vi "helper-snapshot.vi"(11 "RIO List":cluster{"Address":u8, "Connected":bool}[](array[cluster]) {"Address" format="%02d"}) -> (3 "Snapshot":T1[](array[typedef]) {"Dports" format="%08x"})   [LabVIEW 2024]
uses:
  controls/type-snapshot.ctl
  controls/enumVarCtrlIO.ctl
  controls/enum.io.type.ctl
  controls/enum.io.mode.ctl
  controls/IONode.ctl
  controls/type.address.ctl
  controls/typeXyPoint.ctl
  <vilib>/Utility/error.llb/Clear Errors.vi
  util.environment.vi
  util-address-parser.vi
  util.DO.ToString.vi
  Polymorphics/io.command-builder.vi
  Polymorphics/io.command-builder.DO.vi
  Polymorphics/io.command-builder.AI.vi
  Polymorphics/io.command-builder.DI.vi
  io.frame.vi
  io.visa.vi
  io.responseValidator.vi
  Polymorphics/io.command-parser.DI.vi
  Polymorphics/io.command-parser.AI.vi
  globals/globals-engine.vi
panel:
  in  "IO calib select":string(combo)
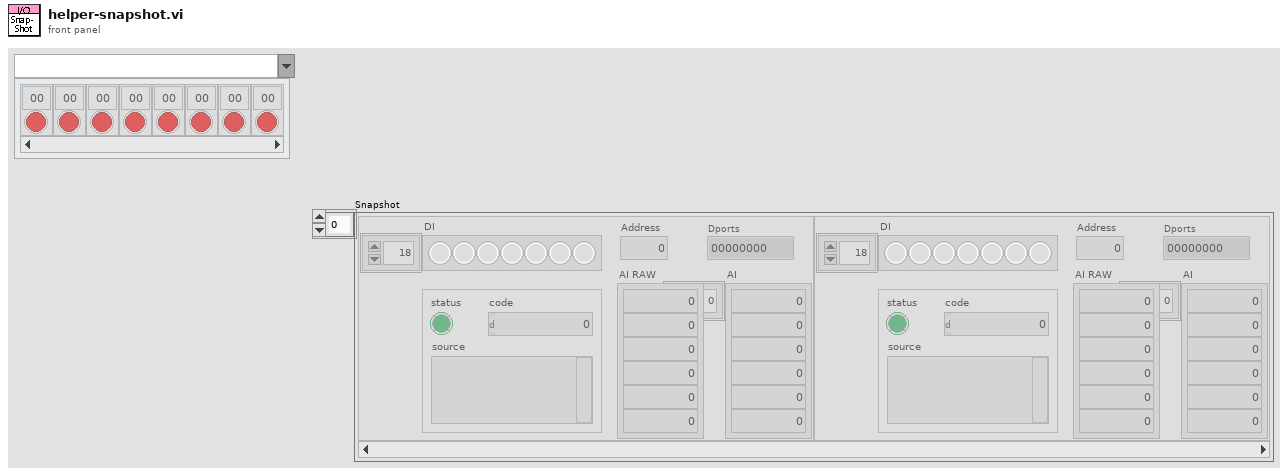
[diagram p1: front panel]
types:
  T1 = typedef "type-snapshot.ctl" = cluster{"Address":u8, "DI":bool[], "status":errorcluster, "AI":dbl[], "Dports":u32, "AI RAW":dbl[]}
  T2 = typedef "enumVarCtrlIO.ctl" = enum16{"IO Get By Key", "IO List Configs", "IO Add By Key", "IO Modify Value By Key", "IO Modify Calib By Key", "IO Modify ADDR By Key", "IO Modify Mode By Key", "IO Modify Type By Key", "IO Modify Name By Key", "IO Remove By Key", "IO Remove All"}
  T3 = typedef "IONode.ctl" = cluster{"ADDR":T4, "Label":string, "Type":T5, "Mode":T6, "Value":string, "Tags":string, "calibration":T7[]}
  T4 = typedef "type.address.ctl" = u16
  T5 = typedef "enum.io.type.ctl" = enum16{"Type", "DI", "DO", "AI", "AO", "VL", "BUF"}
  T6 = typedef "enum.io.mode.ctl" = enum16{"Mode", "RIO", "SIM"}
  T7 = typedef "typeXyPoint.ctl" = cluster{"X":dbl, "Y":dbl}
  T8 = cluster{"Device":u8, "Label":string, "Type":T5, "Mode":T6, "Tags":string}
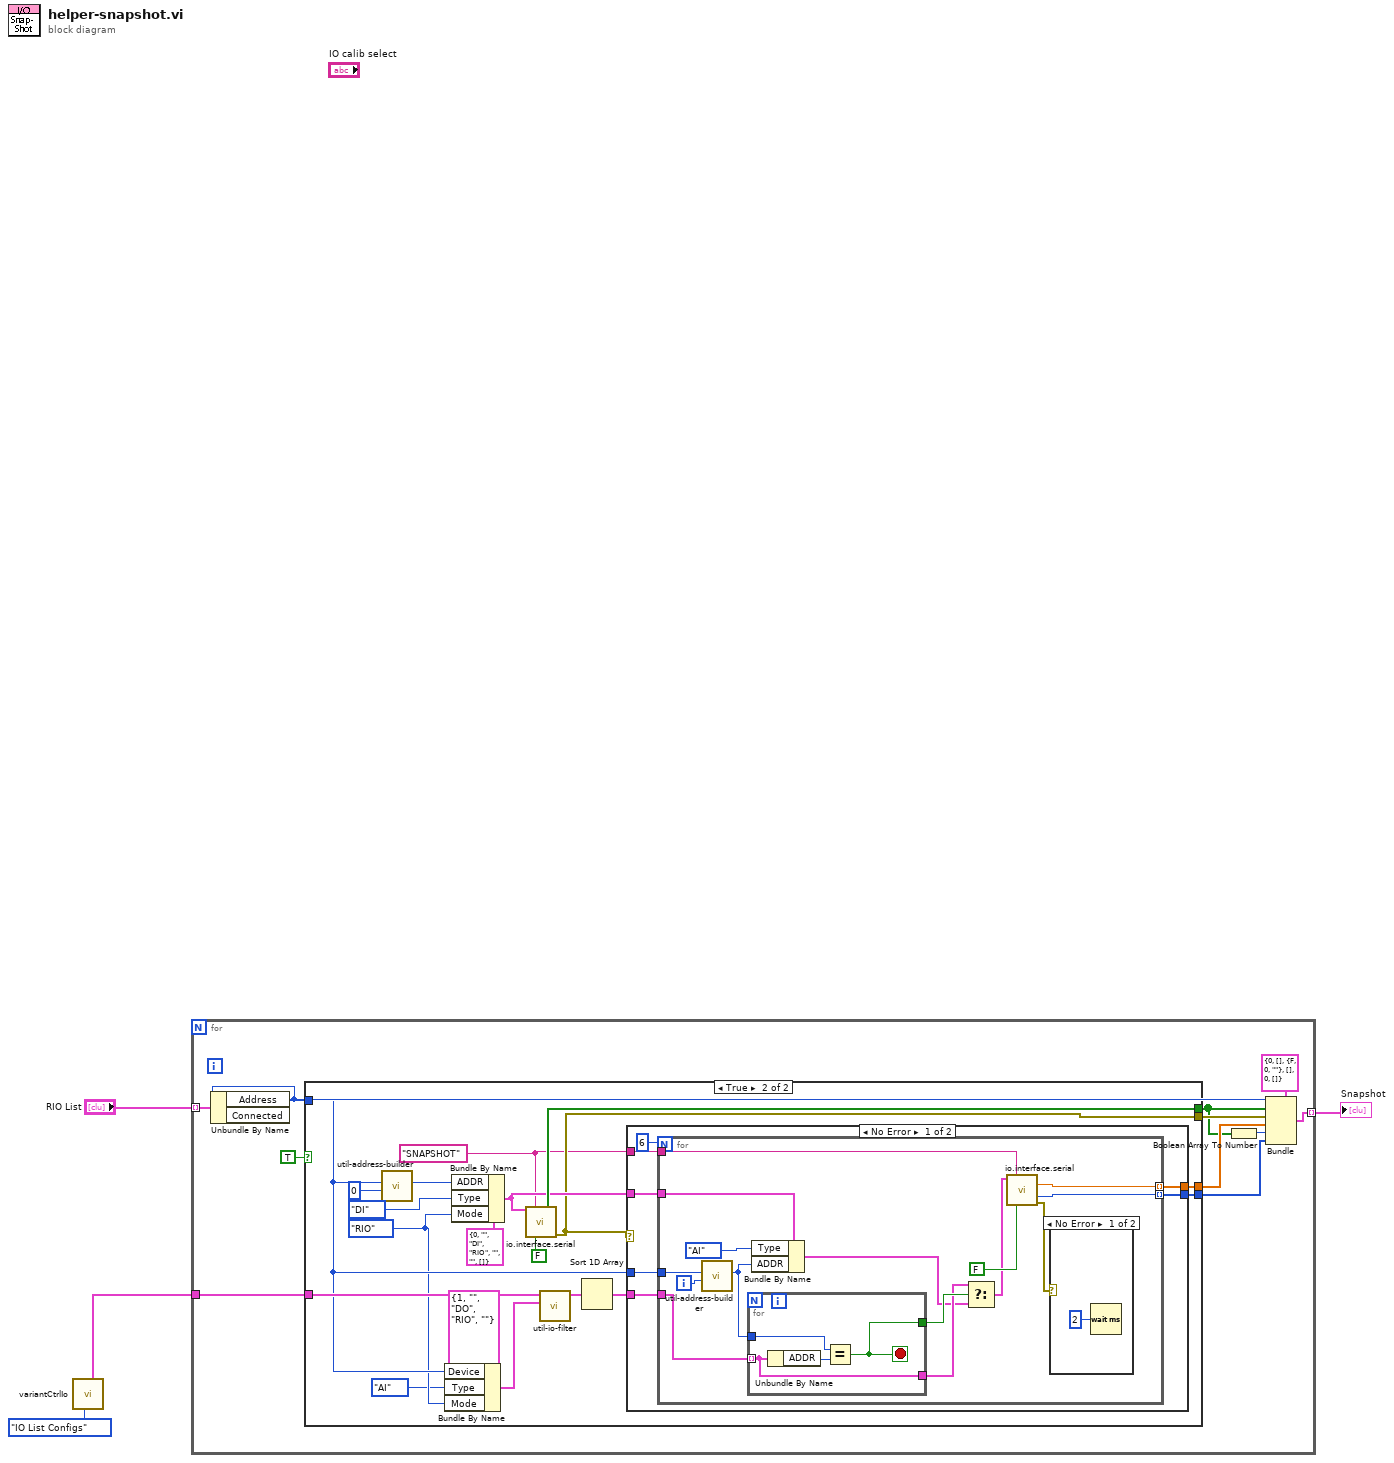
[diagram p0: block diagram]
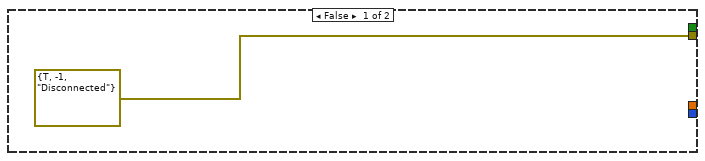
[diagram p2: hidden frame]
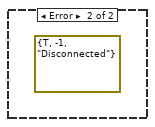
[diagram p4: hidden frame]
diagram:
  n1 = call "variantCtrlIo.vi"("menu (Get Param)"=enumVarCtrlIO."IO List Configs") -> ("IO Configs List"=w1:T3[])  [unwired: 6 in, 4 out]
  n2 = for {
    tunnel: [w15] -> w4 mode=indexing
    tunnel: "RIO List" -> [w12] mode=indexing
    tunnel: w1 -> [w10]
    n3 = Unbundle By Name(w12) -> ("Address"=w11:u8)  [unwired: 1 out]
    n4 = case shown="True" TRUE {
      tunnel: [_ w34] -> w8
      tunnel: [_ w31] -> w14
      tunnel: [errorcluster {"status"=TRUE, "code"=-1, "source"="Disconnected"} ("error out") w19] -> w13
      tunnel: w11 -> [_ w24]
      tunnel: w10 -> [_ w27]
      tunnel: [_ w17] -> w5
      frame False {
      }
      frame True {
        w18 = "SNAPSHOT" ("Caller")
        w23 = enum.io.mode."RIO" ("Mode")
        n5 = call "util-address-builder.vi"("Channel"=u8 0, "Device"=w24) -> ("ADDR"=w30:T4)  [unwired: 9 in]
        n6 = Bundle By Name(cluster=T8 {"Device"=1, "Label"="", "Type"=enum."DO", "Mode"=enum."RIO", "Tags"=""} ("IO Search Conf"), "Device"=w24, "Type"=enum.io.type."AI", "Mode"=w23) -> (w25:T8)
        n7 = Bundle By Name(cluster=T3 {"ADDR"=0, "Label"="", "Type"=enum."DI", "Mode"=enum."RIO", "Value"="", "Tags"="", "calibration"=[]} ("IoConf in"), "ADDR"=w30, "Type"=enum.io.type."DI", "Mode"=w23) -> (w32:T3)
        n8 = call "io.interface.serial.vi"("IoConf in"=w32, "Caller"=w18, "Save to IO Reg(T)"=FALSE) -> ("DI"=w34:bool[], "error out"=w19:errorcluster)  [unwired: 7 in, 4 out]
        n9 = call "util-io-filter.vi"("IO Search Conf"=w25, "IO Configs List"=w27) -> ("Search Results"=w21:T3[])  [unwired: 9 in]
        n10 = Sort 1D Array(array=w21) -> (sorted array=w20:T3[])
        n11 = case shown="No Error" w19 {
          tunnel: w32 -> [w42 _]
          tunnel: [w40 _] -> w31
          tunnel: w24 -> [w39 _]
          tunnel: w20 -> [w38 _]
          tunnel: w18 -> [w37 _]
          tunnel: [w36 _] -> w17
          frame No Error {
            n12 = for {
              N: 6 -> [_]
              tunnel: w42 -> [w57]
              tunnel: w39 -> [w52]
              tunnel: [w55] -> w40 mode=indexing
              tunnel: w38 -> [w51]
              tunnel: w37 -> [w45]
              tunnel: [w44] -> w36 mode=indexing
              i -> [w56]
              n13 = call "util-address-builder.vi"("Channel"=w56, "Device"=w52) -> ("ADDR"=w50:T4)  [unwired: 9 in]
              n14 = for {
                tunnel: w51 -> [w59] mode=indexing
                tunnel: w50 -> [w61]
                tunnel: [w60] -> w49
                tunnel: [w59] -> w48
                stop <- w60 stop-if-true
                n15 = Unbundle By Name(w59) -> ("ADDR"=w62:T4)
                n16 = Equal?(x=w61, y=w62) -> (x = y?=w60:bool)
              }
              n17 = Bundle By Name(cluster=w57, "Type"=enum.io.type."AI", "ADDR"=w50) -> (w47:T3)
              n18 = Select(t=w48, s=w49, f=w47) -> (s? t:f=w46:T3)
              n19 = call "io.interface.serial.vi"("IoConf in"=w46, "Caller"=w45, "Save to IO Reg(T)"=FALSE) -> ("IN (calib)"=w55:dbl, "IN (uncalib)"=w44:u16, "error out"=w43:errorcluster)  [unwired: 7 in, 3 out]
              n20 = case shown="No Error" w43 {
                frame No Error {
                  n21 = Wait (ms)(milliseconds to wait=u32 2) -> ()  [unwired: 1 out]
                }
                frame Error {
                }
              }
            }
          }
          frame Error {
            (unwired) errorcluster {"status"=TRUE, "code"=-1, "source"="Disconnected"} ("error out")
          }
        }
      }
    }
    n22 = Boolean Array To Number(Boolean array=w8) -> (number=w6:u32)
    n23 = Bundle(cluster=T1 {"Address"=0, "DI"=[], "status"={"status"=FALSE, "code"=0, "source"=""}, "AI"=[], "Dports"=0, "AI RAW"=[]} ("Cluster"), "Address"=w11, "DI"=w8, "status"=w13, "AI"=w14, "Dports"=w6, "AI RAW"=w5) -> (w15:T1)
  }
  "Snapshot" <- w4
